vi "App - RUS scan V2.vi"(0 "Lock-in DAQ settings":T5={"Lockin mode"=enum."NI-DAQ", "DAQmx Device"="Dev2", "SR Lockin"="GPIB0::10::INSTR", "Clock Multiplier"=64, "Low-pass filter"=enum."No filtering", "Ranges and couplings "=[{"Range"=2.5, "Coupling"=10106}], "Samples per read"=20, "Record IF"=FALSE, "Auto-phase"=FALSE} {"Ranges and couplings"."Coupling" items=["default"=-1, "RSE"=10083, "NRSE"=10078, "Differential"=10106, "Pseudodifferential"=12529]}, 1 "Save data settings":T6={"Save data"=TRUE, "Data Root Path"=path "D:/Technique/RUS/CeCu2Si2/A116/2_cooling", "File Prefix"="28.49800K_100_3000_0.51000V_0.00000T_Dec19-2014__14-14-48_", "File Format"=enum."BINARY", "Save column names"=FALSE, "File Comments"="\r\nColumns:Frequency\\tX\\tY\r\n    ITC Temp= 299.200000\r\n    LTC Temp= 0.000000\r\n          ITC_set=295.00000\r\n", "User/Prj"="<User Name/Project Description>"}, 5 "temperature":dbl=28.498, 7 "sweep settings":T1={"time gap (min) "=0.0, "Bypass error dialog"=TRUE, "range factor"=1.2, "min gamma(kHz)"=0.005, "max step(Hz)"=1500.0, "min step(Hz)"=0.001, "save freq units"=enum."kHz", "Zero signal?"=FALSE, "time in Gamma --OK"=TRUE, "scan mode"=enum."peak position is known", "power control mode "=enum."none", "time-in-gamma mode"=enum."same for all"}, 9 "Fast swep settings":T4={"Update rate (Hz)"=200.0, "Start F, Hz"=100000.0, "Stop F"=3000000.0, "Number of points"=11520, "Amplitude"=0.51, "Init&amplitude"=TRUE, "IF"=1000.0, "Time constant"=0.001} {"IF" format="%#_6p"; "Amplitude" min=0.0 max=2.5; "Number of points" format="%.0p"; "Stop F" format="%#_6p"; "Start F, Hz" format="%#_6p"; "Update rate (Hz)" format="%0.2f"}, 11 "error in (no error)":errorcluster) -> (6 "Actual file path":path=path "D:/Technique/RUS/CeCu2Si2/A116/2_cooling/December_2014/121914/28.49900K_100_3000_0.51000V_0.00000T_Dec19-2014__14-13-48_001_121914.bin", 15 "error out":errorcluster)   [LabVIEW 2015]
uses:
  RUS/Controls/Sweep settings.ctl
  File/Controls/Save data settings.ctl
  File/Controls/File formats.ctl
  RUS/Controls/Lock-in DAQ settings.ctl
  single sweep - frequency chunks.ctl
  single sweep - adaptive parameters.ctl
  next chunk -- parameters.ctl
  time in gamma mode control.ctl
  find peak -- parameters.ctl
  wavepacket.ctl
  adaptive sweep UI controls.ctl
  next chunk -- algorithm.ctl
  cursor action.ctl
  four-corner circle transformation.ctl
  circle corners.ctl
  next chunk -- action.ctl
  <vilib>/Utility/error.llb/DialogType.ctl
  circle center from three points.vi
  draw a line.vi
  draw a circle.vi
  peak -- guess at omega -- dzdomega.vi
  tale of three indices.vi
  Q -- check range -- i -- real.vi
  filter -- window span logic.vi
  linear interp iiii- complex - z-omega - divide.vi
  linear interpolation iiii- complex.vi
  containing bix.vi
  generate linear region.vi
  peak -- z center from mult phase points.vi
  peak -- estimate for lorentzian.vi
  peak -- fake phase around center.vi
  peak -- get weights.vi
  peak - fit phase around center - V1.vi
  command stack.vi
  tale of three indices -- check state.vi
  Q -- check range -- i -- integer.vi
  Q - not nan -- real.vi
  linear interp iiii- complex - z-omega.vi
  line -- complex.vi
  <vilib>/Utility/error.llb/Clear Errors.vi
  Q - not nan -- integer.vi
  <vilib>/Analysis/baseanly.llb/A x B.vi
  <vilib>/Analysis/baseanly.llb/Complex A x B.vi
  <vilib>/Analysis/Matrix/Numeric/Conversions/Array To Matrix.vi
  <vilib>/Analysis/Matrix/Numeric/Conversions/Array To Matrix - RA2.vi
  <vilib>/Analysis/baseanly.llb/Inverse Matrix.vi
  <vilib>/Analysis/baseanly.llb/Real Inverse Matrix.vi
  array - generate range.vi
  peak -- fit function -- arctan.vi
  <vilib>/gmath/NumericalOptimization/Nonlinear Curve Fit.vi
  <vilib>/gmath/NumericalOptimization/Nonlinear Curve Fit LM.vi
  <resource>/objmgr/daqmx.rc
panel:
  in  "Tab : everything":enum32{"main", "everything else", "adaptive"}(tab)
  out "near omega (kHz)":dbl=50.0
  in  "Subtract a circle?":enum16{"Yes", "No"}(ring)
  in  "complex plane scale gauge":dbl(slide)=0.012396748308571648 caption="Volts" scale=0.0001..0.5
  in  "show plot pallets":bool
  in  "highlight last # sec":dbl=5.0
  out "Plot:response":cluster{dbl[], dbl[]}[](graph)=[{array[11520 elements], array[7540 elements]}, {array[11520 elements], array[7540 elements]}, {[645.57463, 645.57463], [-0.001, 0.001]}, {[769.523, 769.523], [-0.001, 0.001]}, {[1172.39758, 1172.39758], [-0.001, 0.001]}, {[1206.75312, 1206.75312], [-0.001, 0.001]}, {[1510.64651, 1510.64651], [-0.001, 0.001]}, {[1631.67457, 1631.67457], [-0.001, 0.001]}, {[2096.82648, 2096.82648], [-0.001, 0.001]}, {[2105.06377, 2105.06377], [-0.001, 0.001]}, {[2334.70001, 2334.70001], [-0.001, 0.001]}, {[2555.28377, 2555.28377], [-0.001, 0.001]}, {[2670.63046, 2670.63046], [-0.001, 0.001]}, {[2769.74725, 2769.74725], [-0.001, 0.001]}, {[2846.85386, 2846.85386], [-0.001, 0.001]}, {[2876.29657, 2876.29657], [-0.001, 0.001]}, {[2968.3015, 2968.3015], [-0.001, 0.001]}, {[2979.55486, 2979.55486], [-0.001, 0.001]}]
  out "Plot:complex plane":cluster{dbl[], dbl[]}[](graph)=[{array[7540 elements], array[7540 elements]}, {array[1000 elements], array[1000 elements]}, {[0.005000003045536789, 0.004940547817909086, 0.004763119779482496, 0.004470517076413378, 0.004067354228121515, 0.0035599893535622827, 0.0029564238998925634, 0.0022661764548692546, 0.0015001326330342118, 0.0006703734030701707, -0.00021001543629219814, -0.0011271496271373508, -0.0020665654154062474, -0.003013447652938098, -0.003952863441206996, -0.004869997632052148, -0.005750386471414516, -0.0065801457013785584, -0.0073461895232136, -0.008036436968236908, -0.008640002421906627, -0.009147367296465859, -0.009550530144757723, -0.00984313284782684, -0.010020560886253431, -0.010080016113881134, -0.010020560886253431, -0.00984313284782684, -0.009550530144757721, -0.009147367296465859, -0.008640002421906625, -0.008036436968236908, -0.007346189523213599, -0.006580145701378555, -0.005750386471414511, -0.004869997632052148, -0.003952863441206995, -0.0030134476529380966, -0.0020665654154062444, -0.0011271496271373462, -0.00021001543629219988, 0.0006703734030701703, 0.0015001326330342135, 0.0022661764548692572, 0.002956423899892566, 0.0035599893535622853, 0.004067354228121515, 0.004470517076413378, 0.004763119779482496, 0.004940547817909086], [0.00047076259399639255, 0.0014157763757271474, 0.0023458867255961384, 0.0032464252477649408, 0.004103189911783316, 0.004902669027093289, 0.0056322543304607505, 0.00628043982581846, 0.006837003240697381, 0.007293167237570003, 0.007641737837706482, 0.007877217874516685, 0.007995893687151154, 0.007995893687151154, 0.007877217874516684, 0.007641737837706482, 0.0072931672375700024, 0.00683700324069738, 0.00628043982581846, 0.005632254330460749, 0.0049026690270932895, 0.004103189911783315, 0.003246425247764939, 0.002345886725596139, 0.0014157763757271461, 0.0004707625939963901, -0.00047425118773436253, -0.0014043615376033549, -0.0023049000597721585, -0.0031616647237905308, -0.0039611438391005055, -0.004690729142467966, -0.005338914637825676, -0.005895478052704598, -0.00635164204957722, -0.0067002126497136974, -0.0069356926865239, -0.007054368499158369, -0.007054368499158369, -0.006935692686523899, -0.006700212649713698, -0.006351642049577218, -0.005895478052704595, -0.0053389146378256735, -0.004690729142467962, -0.0039611438391004995, -0.0031616647237905303, -0.002304900059772155, -0.001404361537603351, -0.00047425118773435874]}, {[-0.0036773228927567273, -0.003563591256898272, -0.0034498596210398164, -0.003336127985181361, -0.0032223963493229054, -0.0031086647134644495, -0.0029949330776059945, -0.0028812014417475386, -0.002767469805889083, -0.0026537381700306277, -0.0025400065341721722, -0.0024262748983137168, -0.0023125432624552613, -0.002198811626596806, -0.00208507999073835, -0.001971348354879895, -0.0018576167190214393, -0.0017438850831629838, -0.0016301534473045281, -0.0015164218114460727], [0.00792450366560593, 0.007179129558444975, 0.006433755451284022, 0.005688381344123069, 0.004943007236962115, 0.004197633129801161, 0.0034522590226402083, 0.0027068849154792546, 0.001961510808318301, 0.001216136701157347, 0.0004707625939963933, -0.00027461151316456045, -0.0010199856203255125, -0.0017653597274864662, -0.00251073383464742, -0.0032561079418083737, -0.0040014820489693275, -0.004746856156130281, -0.005492230263291235, -0.006237604370452189]}, {[0.004913734537437363, 0.004168360430276409, 0.003422986323115456, 0.0026776122159545028, 0.001932238108793549, 0.0011868640016325952, 0.00044148989447164236, -0.0003038842126893114, -0.0010492583198502652, -0.001794632427011219, -0.0025400065341721727, -0.0032853806413331264, -0.0040307547484940785, -0.004776128855655032, -0.005521502962815986, -0.00626687706997694, -0.0070122511771378935, -0.007757625284298847, -0.008502999391459801, -0.009248373498620755], [0.0016080789525809475, 0.001494347316722492, 0.0013806156808640366, 0.001266884045005581, 0.0011531524091471254, 0.00103942077328867, 0.0009256891374302145, 0.0008119575015717589, 0.0006982258657133035, 0.0005844942298548479, 0.00047076259399639244, 0.000357030958137937, 0.00024329932227948152, 0.00012956768642102606, 1.5836050562570382e-05, -9.789558529588508e-05, -0.00021162722115434054, -0.000325358857012796, -0.0004390904928712517, -0.0005528221287297071]}]
  in  "progress (sec)":dbl(slide)=47.30199999999604 caption="seconds" min=80.0 max=80.0 scale=0.0..54.0
  in  "Plot when running":bool
  in  "Graph update rate, ms":u32=50
  out "near gamma (kHz)":dbl=50.0
  in  "stop":bool
  out "Progress, %":u8(slide)=82 scale=0.0..100.0
  in  "Tab : sweep controls":enum32{"Main controls", "File", "Advanced"}(tab)
  in  "Manual\nPhase":dbl(slide) scale=-180.0..180.0
  out "Error status byte\n(bit 5 - FAST aborted)":u8 format="%08b"
  out "STD status byte":u8 format="%08b"
  out "DO array  making time":u32
  out "DO write time, ms":u32=23
  out "Loop counter":i32=575
  out "Pre-sweep delay, s":dbl=0.2
  out "Samples in buffer":u32
  out "Actual setup time, ms":u32=1812
  out "line two":cluster{dbl[], dbl[]}={[0.004913734537437363, 0.004168360430276409, 0.003422986323115456, 0.0026776122159545028, 0.001932238108793549, 0.0011868640016325952, 0.00044148989447164236, -0.0003038842126893114, -0.0010492583198502652, -0.001794632427011219, -0.0025400065341721727, -0.0032853806413331264, -0.0040307547484940785, -0.004776128855655032, -0.005521502962815986, -0.00626687706997694, -0.0070122511771378935, -0.007757625284298847, -0.008502999391459801, -0.009248373498620755], [0.0016080789525809475, 0.001494347316722492, 0.0013806156808640366, 0.001266884045005581, 0.0011531524091471254, 0.00103942077328867, 0.0009256891374302145, 0.0008119575015717589, 0.0006982258657133035, 0.0005844942298548479, 0.00047076259399639244, 0.000357030958137937, 0.00024329932227948152, 0.00012956768642102606, 1.5836050562570382e-05, -9.789558529588508e-05, -0.00021162722115434054, -0.000325358857012796, -0.0004390904928712517, -0.0005528221287297071]}
  out "circle":cluster{dbl[], dbl[]}={[0.005000003045536789, 0.004940547817909086, 0.004763119779482496, 0.004470517076413378, 0.004067354228121515, 0.0035599893535622827, 0.0029564238998925634, 0.0022661764548692546, 0.0015001326330342118, 0.0006703734030701707, -0.00021001543629219814, -0.0011271496271373508, -0.0020665654154062474, -0.003013447652938098, -0.003952863441206996, -0.004869997632052148, -0.005750386471414516, -0.0065801457013785584, -0.0073461895232136, -0.008036436968236908, -0.008640002421906627, -0.009147367296465859, -0.009550530144757723, -0.00984313284782684, -0.010020560886253431, -0.010080016113881134, -0.010020560886253431, -0.00984313284782684, -0.009550530144757721, -0.009147367296465859, -0.008640002421906625, -0.008036436968236908, -0.007346189523213599, -0.006580145701378555, -0.005750386471414511, -0.004869997632052148, -0.003952863441206995, -0.0030134476529380966, -0.0020665654154062444, -0.0011271496271373462, -0.00021001543629219988, 0.0006703734030701703, 0.0015001326330342135, 0.0022661764548692572, 0.002956423899892566, 0.0035599893535622853, 0.004067354228121515, 0.004470517076413378, 0.004763119779482496, 0.004940547817909086], [0.00047076259399639255, 0.0014157763757271474, 0.0023458867255961384, 0.0032464252477649408, 0.004103189911783316, 0.004902669027093289, 0.0056322543304607505, 0.00628043982581846, 0.006837003240697381, 0.007293167237570003, 0.007641737837706482, 0.007877217874516685, 0.007995893687151154, 0.007995893687151154, 0.007877217874516684, 0.007641737837706482, 0.0072931672375700024, 0.00683700324069738, 0.00628043982581846, 0.005632254330460749, 0.0049026690270932895, 0.004103189911783315, 0.003246425247764939, 0.002345886725596139, 0.0014157763757271461, 0.0004707625939963901, -0.00047425118773436253, -0.0014043615376033549, -0.0023049000597721585, -0.0031616647237905308, -0.0039611438391005055, -0.004690729142467966, -0.005338914637825676, -0.005895478052704598, -0.00635164204957722, -0.0067002126497136974, -0.0069356926865239, -0.007054368499158369, -0.007054368499158369, -0.006935692686523899, -0.006700212649713698, -0.006351642049577218, -0.005895478052704595, -0.0053389146378256735, -0.004690729142467962, -0.0039611438391004995, -0.0031616647237905303, -0.002304900059772155, -0.001404361537603351, -0.00047425118773435874]}
  out "line one":cluster{dbl[], dbl[]}={[-0.0036773228927567273, -0.003563591256898272, -0.0034498596210398164, -0.003336127985181361, -0.0032223963493229054, -0.0031086647134644495, -0.0029949330776059945, -0.0028812014417475386, -0.002767469805889083, -0.0026537381700306277, -0.0025400065341721722, -0.0024262748983137168, -0.0023125432624552613, -0.002198811626596806, -0.00208507999073835, -0.001971348354879895, -0.0018576167190214393, -0.0017438850831629838, -0.0016301534473045281, -0.0015164218114460727], [0.00792450366560593, 0.007179129558444975, 0.006433755451284022, 0.005688381344123069, 0.004943007236962115, 0.004197633129801161, 0.0034522590226402083, 0.0027068849154792546, 0.001961510808318301, 0.001216136701157347, 0.0004707625939963933, -0.00027461151316456045, -0.0010199856203255125, -0.0017653597274864662, -0.00251073383464742, -0.0032561079418083737, -0.0040014820489693275, -0.004746856156130281, -0.005492230263291235, -0.006237604370452189]}
  out "frequency":dbl[](array[numeric])
  out "complex data":cdb[](array[numeric])
  out "#data points so far":i32=9480
  out "last data":cdb[](array[numeric])=[-0.0013862457351888618+0.00908142415858101i, -0.0013023312189548073+0.009148157349497919i, -0.001321430292511047+0.009061460065413475i, -0.001363391573336929+0.009045433130201685i, -0.001296708698532554+0.009000112664646402i, -0.0013667002669505222+0.009050113974772414i, -0.0012817676519993981+0.009066319936344113i, -0.0013424252885312644+0.008962242292230364i, -0.0014137356567434898+0.009049299475543717i, -0.0012869072704579012+0.00899110197613083i, -0.0013910227339383506+0.009040086299077377i, -0.0013472731057654439+0.009083303189564951i, -0.001381966900473036+0.009046535653865845i, -0.0013652417984066345+0.009101756771060749i, -0.0013461643267386587+0.008999329508834603i, -0.0013471376638622685+0.009069385579497309i, -0.0013236258377476435+0.009072036195700378i, -0.0013196021377368792+0.009075087400102249i, -0.0013182324903640112+0.009113697088335707i, -0.0012918150838322992+0.009064845988581937i]
  out "fancy circles":cluster{dbl[], dbl[]}[](array[cluster])
  out "fancy lines":cluster{dbl[], dbl[]}[](array[cluster])=[{[645.57463, 645.57463], [-0.001, 0.001]}, {[769.523, 769.523], [-0.001, 0.001]}, {[1172.39758, 1172.39758], [-0.001, 0.001]}, {[1206.75312, 1206.75312], [-0.001, 0.001]}, {[1510.64651, 1510.64651], [-0.001, 0.001]}, {[1631.67457, 1631.67457], [-0.001, 0.001]}, {[2096.82648, 2096.82648], [-0.001, 0.001]}, {[2105.06377, 2105.06377], [-0.001, 0.001]}, {[2334.70001, 2334.70001], [-0.001, 0.001]}, {[2555.28377, 2555.28377], [-0.001, 0.001]}, {[2670.63046, 2670.63046], [-0.001, 0.001]}, {[2769.74725, 2769.74725], [-0.001, 0.001]}, {[2846.85386, 2846.85386], [-0.001, 0.001]}, {[2876.29657, 2876.29657], [-0.001, 0.001]}, {[2968.3015, 2968.3015], [-0.001, 0.001]}, {[2979.55486, 2979.55486], [-0.001, 0.001]}]
  in  "adaptive state":T8={"peaks are known -- parameters"={"Def Gamma (kHz)"=10.0, "dV"=17.0, "time in Gamma (sec)"=3.0, "phi-star"=0.0, "all peaks (kHz)"=[645.57463, 769.523, 1172.39758, 1206.75312, 1510.64651, 1631.67457, 2096.82648, 2105.06377, 2334.70001, 2555.28377, 2670.63046, 2769.74725, 2846.85386, 2876.29657, 2968.3015, 2979.55486], "delta t (sec)"=0.005, "default step (Hz)"=251.73611111111111, "all gamma (kHz)"=[0.05963, 1.26052, 0.07474, 0.14496, 0.02522, 0.0921, 0.08571, 0.32008, 0.01, 0.00491, 2.14403, 0.17331, 7.48912, 0.20157, 0.17918, 0.145], "peaks OK"=TRUE, "gamma OK"=TRUE, "near omega (kHz)"=0.0, "near gamma (kHz)"=0.0, "min step (Hz)"=0.001, "max step(Hz)"=1500.0, "min gamma (kHz)"=0.005, "all time in gamma (sec)"=[], "time in gamma OK"=FALSE, "time-in-gamma mode"=enum."same for all"}, "find peak - parameters"={"wavepacket"={"R"=0.5, "wave number"=17.0, "delta k"=7.0, "radii vector"=[], "radial section"=[], "wave vector"=22.0, "wavepacket is"=TRUE}, "number of grid points"=70, "decimation threshold"=1, "Voltage range"=0.1, "target freq step"=20.0, "target spot size"=0.05, "factor"=1.0, "another factor"=1.0, "analyze last # sec"=3, "scale factor"=3}} {"find peak - parameters"."wavepacket"."delta k" format="%#_3f"; "find peak - parameters"."wavepacket"."wave number" format="%#_3f"; "find peak - parameters"."wavepacket"."R" format="%#_3f"}
  in  "chunks":T12={"start F (Hz)"=100000.0, "stop F (Hz)"=3000000.0, "total number of points"=11520, "chunk size"=20, "freq step (Hz)"=0.7518687555352066, "update rate (Hz)"=200.0, "adaptive parameters"={"peaks are known -- parameters"={"Def Gamma (kHz)"=10.0, "dV"=17.0, "time in Gamma (sec)"=3.0, "phi-star"=0.0, "all peaks (kHz)"=[645.57463, 769.523, 1172.39758, 1206.75312, 1510.64651, 1631.67457, 2096.82648, 2105.06377, 2334.70001, 2555.28377, 2670.63046, 2769.74725, 2846.85386, 2876.29657, 2968.3015, 2979.55486], "delta t (sec)"=0.005, "default step (Hz)"=251.73611111111111, "all gamma (kHz)"=[0.05963, 1.26052, 0.07474, 0.14496, 0.02522, 0.0921, 0.08571, 0.32008, 0.01, 0.00491, 2.14403, 0.17331, 7.48912, 0.20157, 0.17918, 0.145], "peaks OK"=TRUE, "gamma OK"=TRUE, "near omega (kHz)"=0.0, "near gamma (kHz)"=0.0, "min step (Hz)"=0.001, "max step(Hz)"=1500.0, "min gamma (kHz)"=0.005, "all time in gamma (sec)"=[], "time in gamma OK"=FALSE, "time-in-gamma mode"=enum."same for all"}, "find peak - parameters"={"wavepacket"={"R"=0.5, "wave number"=17.0, "delta k"=7.0, "radii vector"=[], "radial section"=[], "wave vector"=22.0, "wavepacket is"=TRUE}, "number of grid points"=70, "decimation threshold"=1, "Voltage range"=0.1, "target freq step"=20.0, "target spot size"=0.05, "factor"=1.0, "another factor"=1.0, "analyze last # sec"=3, "scale factor"=3}}, "total sweep time (sec)"=57.6, "chunk time (sec)"=0.1, "spot size (V)"=0.0, "uniform freq step (Hz)"=251.73611111111111, "next start freq (Hz)"=2876231.1242983374} {"next start freq (Hz)" format="%#9_8f"; "uniform freq step (Hz)" format="%#_3f"; "spot size (V)" format="%#_2f"; "adaptive parameters"."find peak - parameters"."wavepacket"."delta k" format="%#_3f"; "adaptive parameters"."find peak - parameters"."wavepacket"."wave number" format="%#_3f"; "adaptive parameters"."find peak - parameters"."wavepacket"."R" format="%#_3f"; "freq step (Hz)" format="%#4_4f"; "stop F (Hz)" format="%#_3f"; "start F (Hz)" format="%#_3f"}
  # "SRS Lockin related"
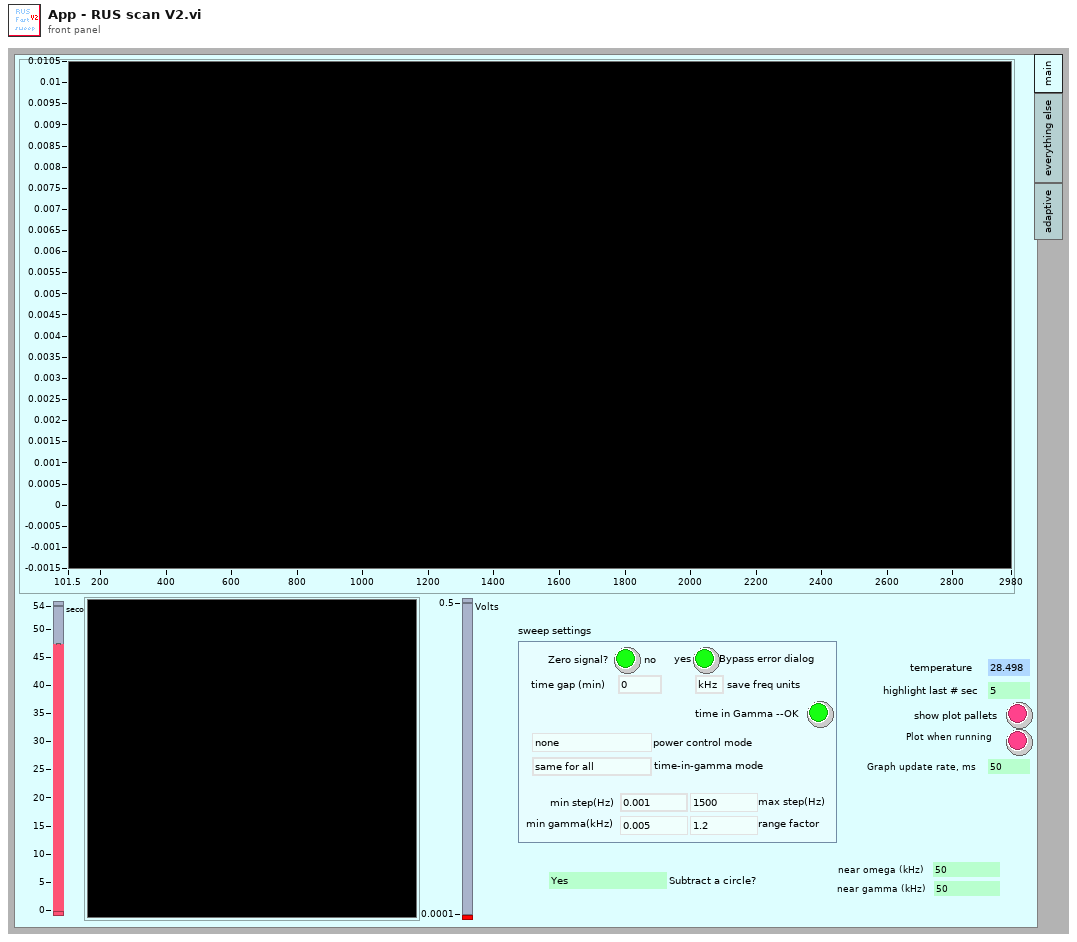
[diagram p1: front panel]
types:
  T1 = typedef "adaptive sweep UI controls.ctl" = cluster{"time gap (min) ":dbl, "Bypass error dialog":bool, "range factor":dbl, "min gamma(kHz)":dbl, "max step(Hz)":dbl, "min step(Hz)":dbl, "save freq units":enum16{"kHz", "Hz"}, "Zero signal?":bool, "time in Gamma --OK":bool, "scan mode":T2, "power control mode ":enum16{"power vs Temp", "power vs Time", "none"}, "time-in-gamma mode":T3}
  T2 = typedef "next chunk -- algorithm.ctl" = enum16{"peak position is known", "uniform", "predictive"}
  T3 = typedef "time in gamma mode control.ctl" = enum16{"same for all", "each one different", "uniform scan"}
  T4 = typedef "Sweep settings.ctl" = cluster{"Update rate (Hz)":dbl, "Start F, Hz":dbl, "Stop F":dbl, "Number of points":i32, "Amplitude":dbl, "Init&amplitude":bool, "IF":dbl, "Time constant":dbl}
  T5 = typedef "Lock-in DAQ settings.ctl" = cluster{"Lockin mode":enum16{"SRS", "NI-DAQ"}, "DAQmx Device":tag, "SR Lockin":refnum<visa-resource-name>, "Clock Multiplier":i32, "Low-pass filter":enum16{"No filtering", "Butterworth", "Bessel"}, "Ranges and couplings ":cluster{"Range":dbl, "Coupling":i32}[], "Samples per read":i32, "Record IF":bool, "Auto-phase":bool}
  T6 = typedef "Save data settings.ctl" = cluster{"Save data":bool, "Data Root Path":path, "File Prefix":string, "File Format":T7, "Save column names":bool, "File Comments":string, "User/Prj":string}
  T7 = typedef "File formats.ctl" = enum16{"TDMS", "ASCII", "BINARY"}
  T8 = typedef "single sweep - adaptive parameters.ctl" = cluster{"peaks are known -- parameters":T9, "find peak - parameters":T10}
  T9 = typedef "next chunk -- parameters.ctl" = cluster{"Def Gamma (kHz)":dbl, "dV":dbl, "time in Gamma (sec)":dbl, "phi-star":dbl, "all peaks (kHz)":dbl[], "delta t (sec)":dbl, "default step (Hz)":dbl, "all gamma (kHz)":dbl[], "peaks OK":bool, "gamma OK":bool, "near omega (kHz)":dbl, "near gamma (kHz)":dbl, "min step (Hz)":dbl, "max step(Hz)":dbl, "min gamma (kHz)":dbl, "all time in gamma (sec)":dbl[], "time in gamma OK":bool, "time-in-gamma mode":T3}
  T10 = typedef "find peak -- parameters.ctl" = cluster{"wavepacket":T11, "number of grid points":i32, "decimation threshold":i32, "Voltage range":dbl, "target freq step":dbl, "target spot size":dbl, "factor":dbl, "another factor":dbl, "analyze last # sec":i32, "scale factor":i32}
  T11 = typedef "wavepacket.ctl" = cluster{"R":dbl, "wave number":dbl, "delta k":dbl, "radii vector":dbl[], "radial section":cdb[], "wave vector":dbl, "wavepacket is":bool}
  T12 = typedef "single sweep - frequency chunks.ctl" = cluster{"start F (Hz)":dbl, "stop F (Hz)":dbl, "total number of points":i32, "chunk size":i32, "freq step (Hz)":dbl, "update rate (Hz)":dbl, "adaptive parameters":T8, "total sweep time (sec)":dbl, "chunk time (sec)":dbl, "spot size (V)":dbl, "uniform freq step (Hz)":dbl, "next start freq (Hz)":dbl}
  T13 = typedef "RUS settings.ctl" = cluster{"NI-DAQ lockin settings":T14, "Fast swep settings":T4, "Pre-sweep delay, s":dbl, "Lockin mode":enum16{"SRS", "NI-DAQ"}, "SR Lockin":refnum<visa-resource-name>, "DAQmx Device":tag, "Clock Multiplier":i32, "Fast Sweep Data Out":cluster{"DO clock task":refnum<k21>, "DO task":refnum<k21>, "Update clock task":refnum<k21>, "DAQ lockin task":refnum<k21>, "Pre-sweep counter task":refnum<k21>}, "Lockin Range, V":sgl, "F Array":dbl[], "Freq. update clock terminal":string, "DO Clock Rate (Hz)":dbl, "ADC clock terminal":string, "Pre-sweep counter terminal":string, "Samples per read":i32, "DO clock terminal":string, "Pre-sweep points":i32, "F points per write":i32, "Total sweep time, s":dbl, "Initial SYNTH phase":dbl, "Record IF":bool, "Save data settings":T6, "Data file path":path, "New data user event":refnum<user-event>, "Stop user event":refnum<user-event>, "Number of channels":i32, "Auto-phase":bool}
  T14 = typedef "RUS NI-DAQ Lockin Settings.ctl" = cluster{"Samples per sine wave":i32, "Sine waves per freq step":i32, "Output Representation":enum16{"Real/Imaginary", "Polar"}, "Low-pass filter":enum16{"No filtering", "Butterworth", "Bessel"}, "Ranges and couplings ":cluster{"Range":dbl, "Coupling":i32}[]}
  T15 = typedef "next chunk -- action.ctl" = enum16{"empty", "init - uniform", "next chunk - uniform", "next chunk - peaks are known", "init - peaks are known", ""}
  T16 = typedef "circle corners.ctl" = cluster{"z (-pi/2)":cdb, "z(inf)":cdb, "z (pi/2)":cdb, "z center":cdb, "z(0)":cdb, "radius":dbl}
  T17 = typedef "four-corner circle transformation.ctl" = enum16{"z(c) z(inf)", "z(c) z(zero)", "fix phase", "calculate lorentzian", "z(0) z(+-pi/2)", "shift to zcenter"}
  T18 = typedef "cursor action.ctl" = enum16{"range", "read", "write", "check", "zoom out", "smart zoom out"}
  T19 = typedef "DialogType.ctl" = u16
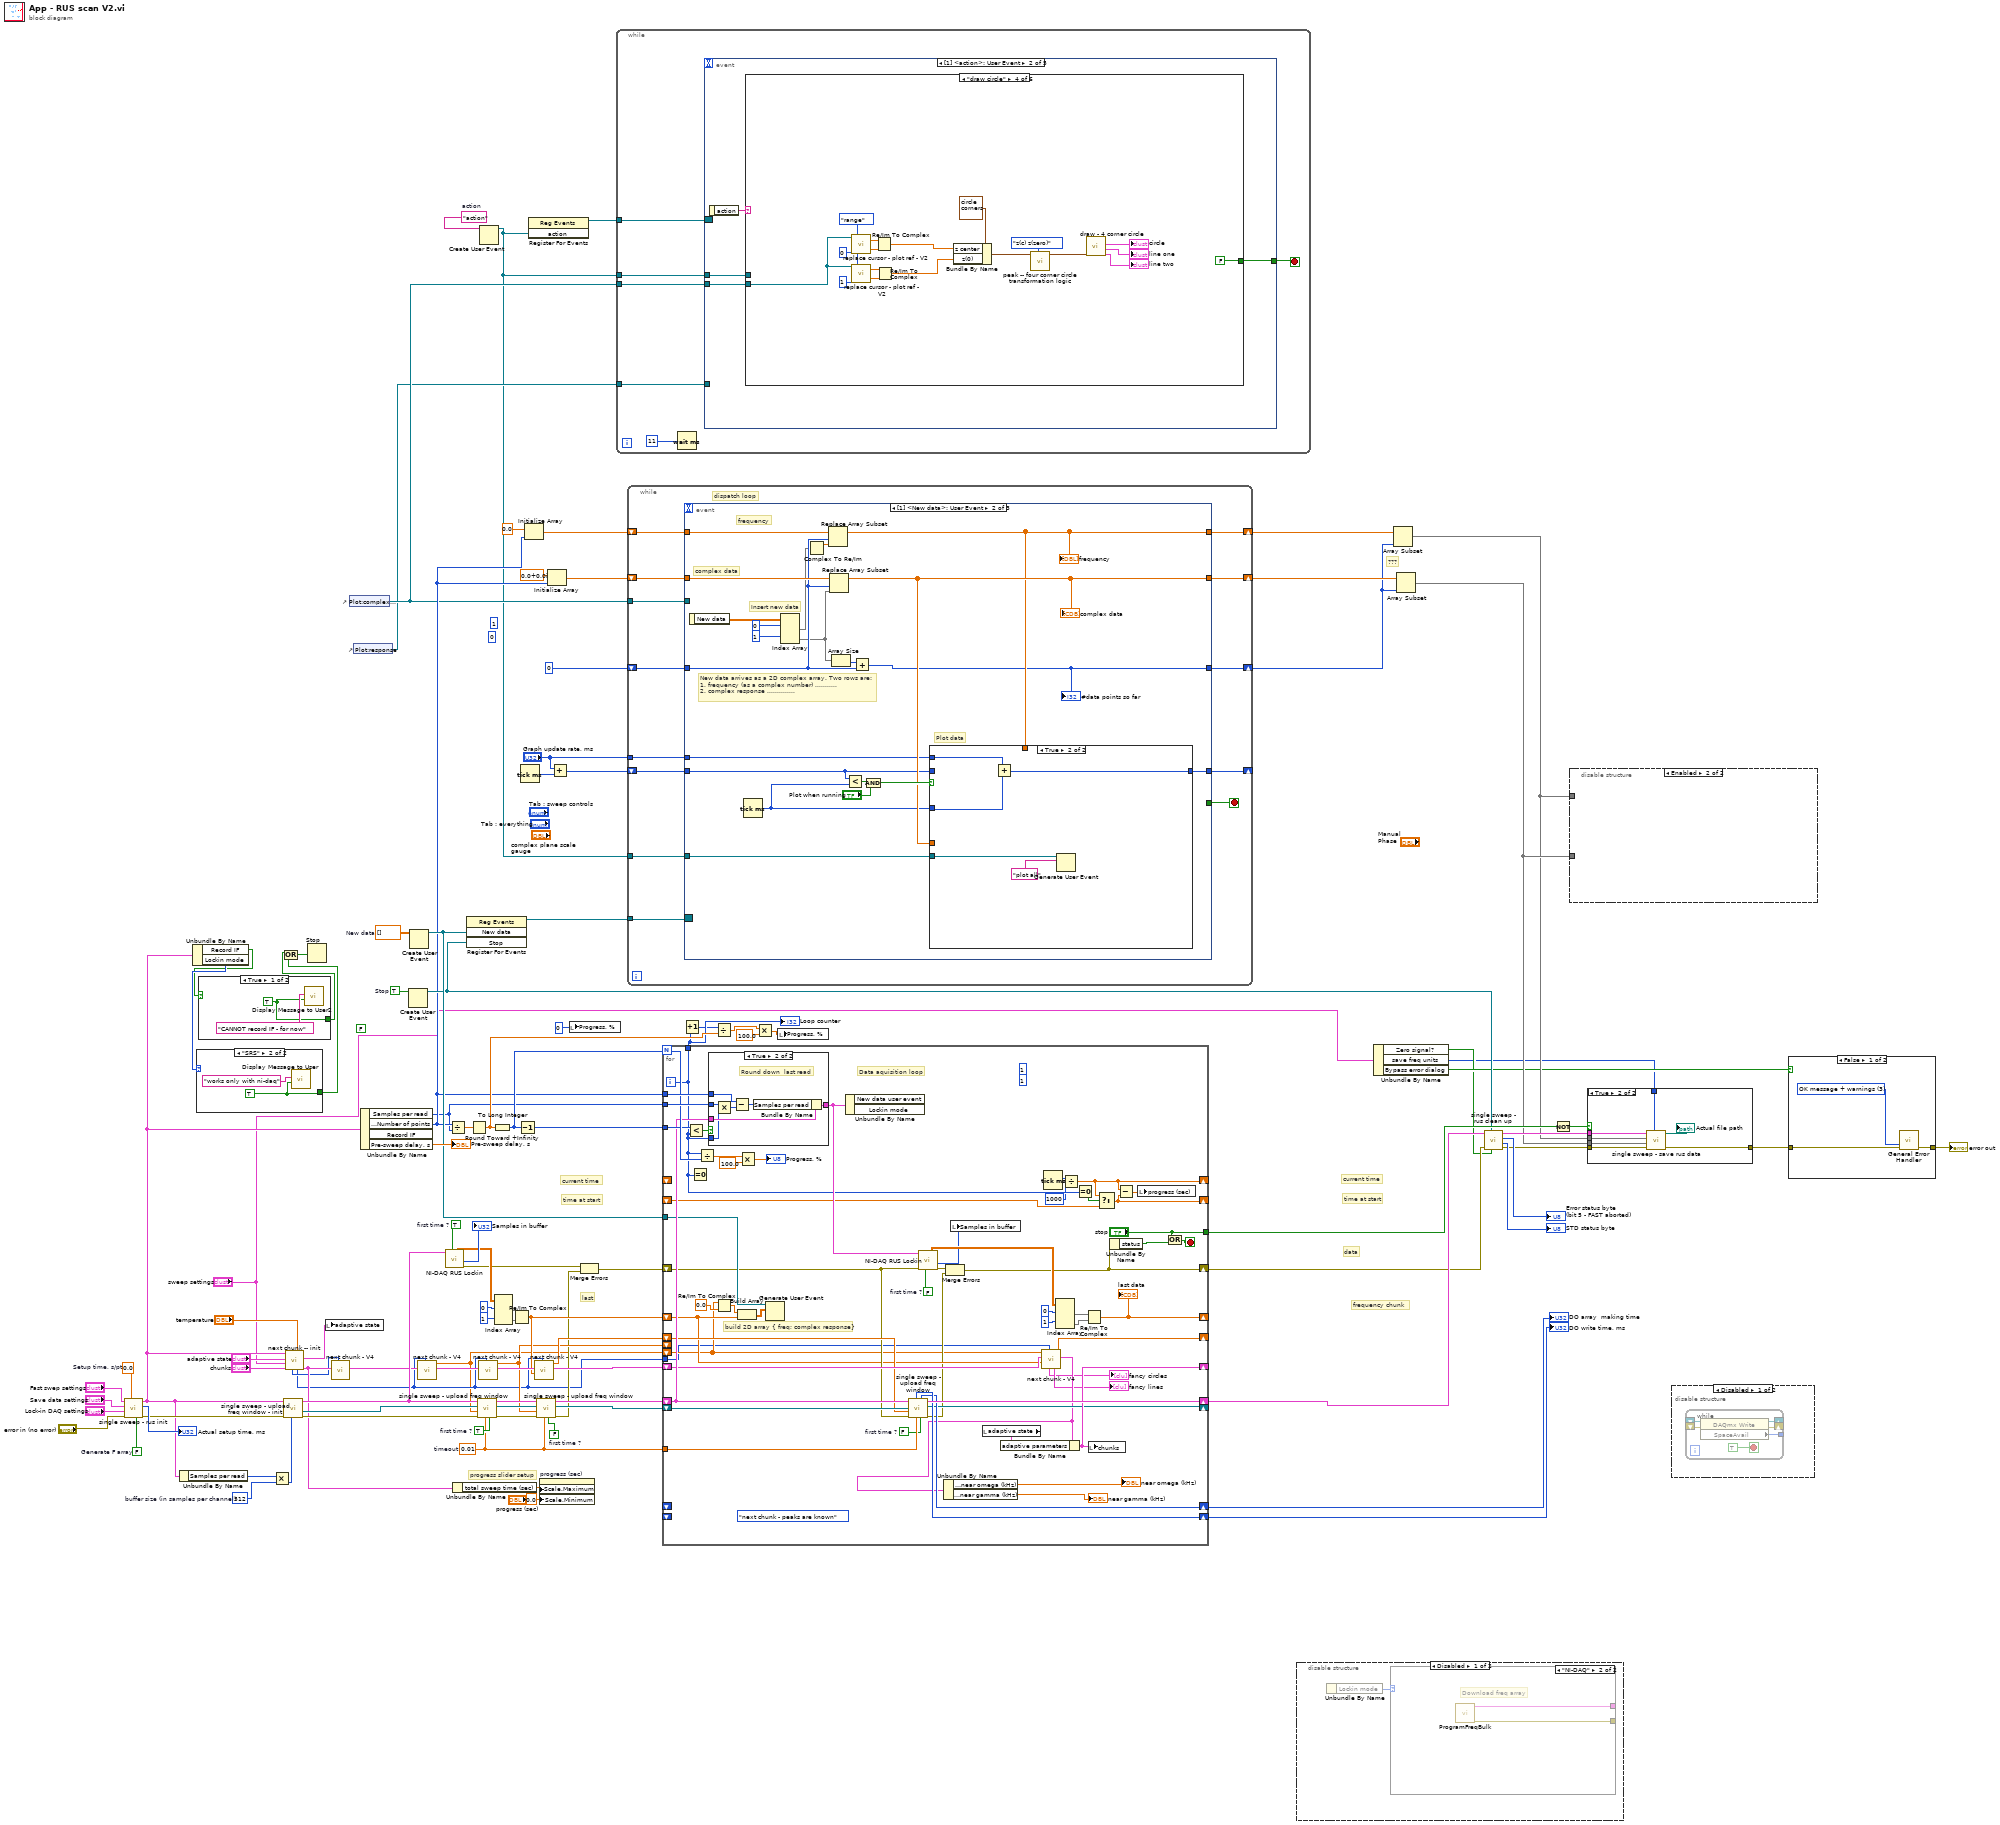
[diagram p0: block diagram]
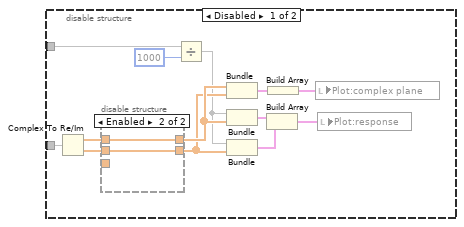
[diagram p2: hidden frame]
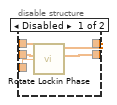
[diagram p3: hidden frame]
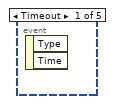
[diagram p4: hidden frame]
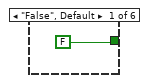
[diagram p5: hidden frame]
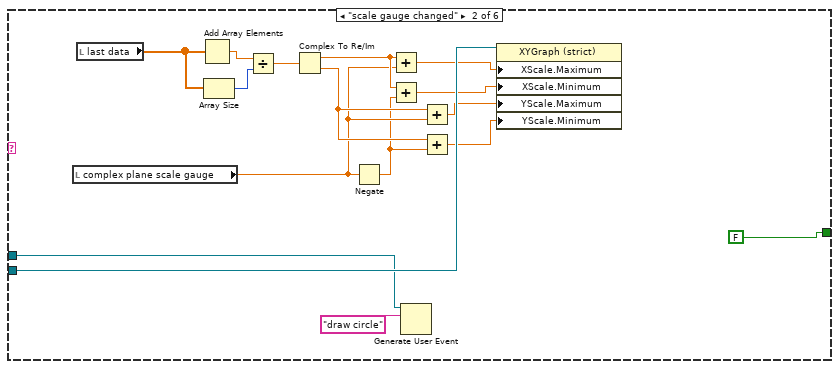
[diagram p6: hidden frame]
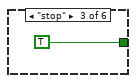
[diagram p7: hidden frame]
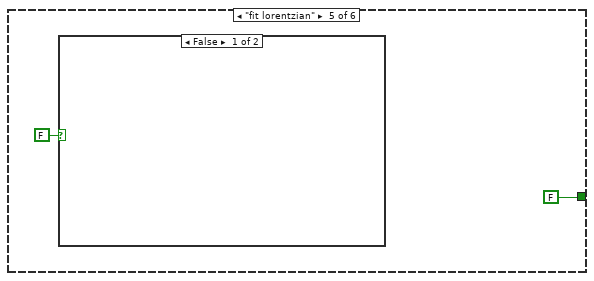
[diagram p8: hidden frame]
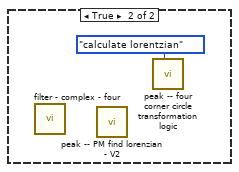
[diagram p9: hidden frame]
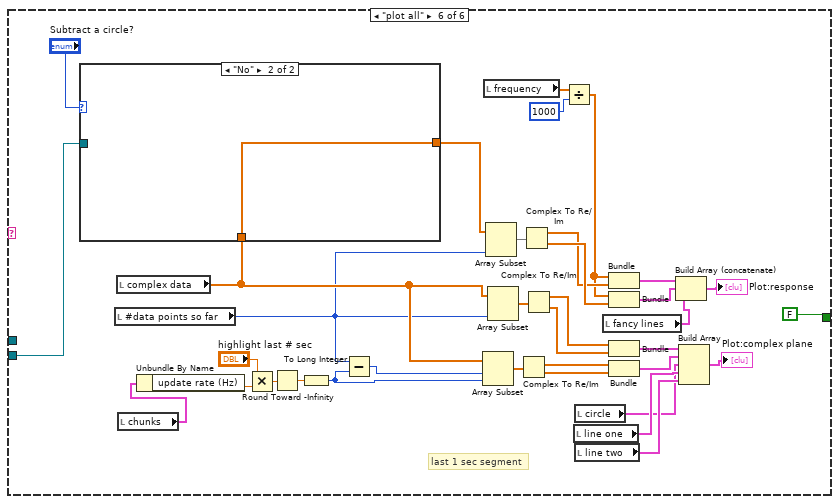
[diagram p10: hidden frame]
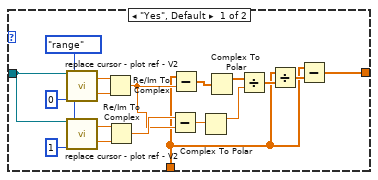
[diagram p11: hidden frame]
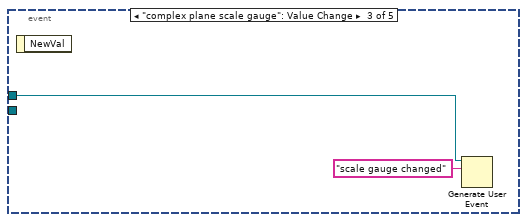
[diagram p12: hidden frame]
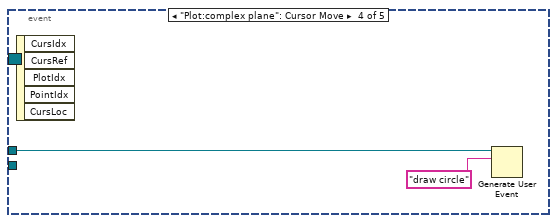
[diagram p13: hidden frame]
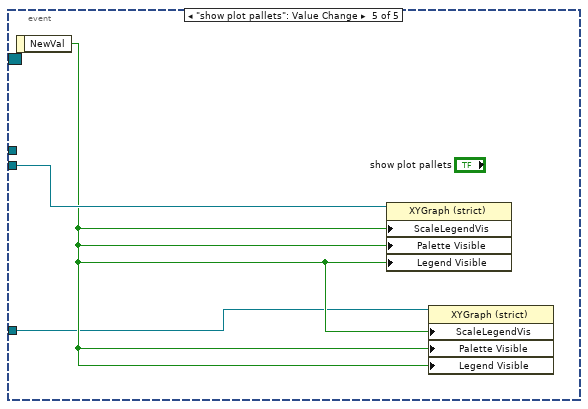
[diagram p14: hidden frame]
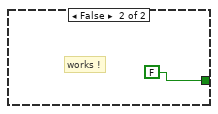
[diagram p16: hidden frame]
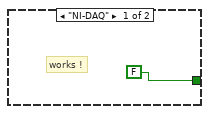
[diagram p17: hidden frame]
diagram:
  w5 = "action"  # action
  w28 = TRUE  # first time ?
  w29 = FALSE  # Generate F array
  w30 = 0.0  # Setup time, s/pt
  w33 = u32 512  # buffer size (in samples per channel)
  w48 = FALSE  # first time ?
  (unwired) 0 ("disabled index (col)")
  (unwired) FALSE
  (unwired) 1 ("dimension size")
  w67 = cdb[][] []  # New data
  w69 = TRUE  # Stop
  w73 = TRUE  # first time ?
  w41 = 0.01  # timeout
  # "data"
  # "frequency chunk"
  # "last"
  # "time at start"
  # "current time"
  # "time at start"
  # "current time"
  # "progress slider setup"
  # "???"
  n1 = call "single sweep - rus init.vi"("Generate F array"=w29, "Setup time, s/pt"=w30, "error in (no error)"="error in (no error)", "Lock-in DAQ settings"="Lock-in DAQ settings", "Save data settings"="Save data settings", "Fast swep settings"="Fast swep settings") -> ("error out"=w76:errorcluster, "Actual setup time, ms"=→"Actual setup time, ms":u32, "RUS settings out"=w18:T13)  [unwired: 2 in, 1 out]
  n2 = Unbundle By Name(w18) -> ("Samples per read"=w31:i32)
  n3 = Unbundle By Name(w18) -> ("Record IF"=w56:bool, "Lockin mode"=w75:enum16{"SRS", "NI-DAQ"})
  n4 = case shown="\"SRS\"" w75 {
    tunnel: [FALSE w108] -> w58
    frame "NI-DAQ" {
      # "works !"
    }
    frame "SRS" {
      w108 = TRUE
      n5 = call "Display Message to User"("Enable"=w108, "Message"="works only with ni-daq") -> ()  [unwired: 8 in, 2 out]
    }
  }
  n6 = case shown="True" w56 {
    tunnel: [w110 FALSE] -> w57
    frame True {
      w110 = TRUE
      n7 = call "Display Message to User2"("Enable"=w110, "Message"="CANNOT record IF - for now") -> ()  [unwired: 8 in, 2 out]
    }
    frame False {
      # "works !"
    }
  }
  n8 = Multiply(x=w31, y=w33) -> (x*y=w32:u32)
  n9 = Or(x=w57, y=w58) -> (x .or. y?=w55:bool)
  n10 = call "single sweep - upload freq window - init.vi"("buffer size (in samples per channel)"=w32, "error in (no error)"=w76, "RUS settings"=w18) -> ("error - out"=w37:errorcluster, "task out"=w74:refnum<k21>, "RUS settings out"=w49:T13)  [unwired: 6 in]
  n11 = call "next chunk -- init.vi"("temperature"="temperature", "chunks"="chunks", "sweep settings"="sweep settings", "adaptive parameters"="adaptive state", "RUS settings"=w18) -> ("chunks out"=w17:T12, "adaptive parameters out"=w15:T8, "next chunk action"=w11:T15, "next chunk init action"=w14:T15)  [unwired: 3 in]
  n12 = Stop(stop? (T)=w55) -> ()
  n13 = local write "adaptive state"(w15) -> ()
  n14 = call "next chunk - V4.vi"("next chunk action"=w14, "chunks"=w17) -> ("chunks out"=w12:T12)  [unwired: 6 in, 3 out]
  n15 = control-ref of="Plot:complex plane"() -> (w3:refnum<vi>)
  n16 = control-ref of="Plot:response"() -> (w2:refnum<vi>)
  n17 = Unbundle By Name(w18) -> ("Samples per read"=w50:i32, "Fast swep settings.Number of points"=w51:i32, "Pre-sweep delay, s"=→"Pre-sweep delay, s":dbl)  [unwired: 1 out]
  n18 = Create User Event(user event datatype=w69) -> (user event=w62:refnum<user-event>)  [unwired: 1 in, 1 out]
  n19 = Create User Event(user event datatype=w67) -> (user event=w68:refnum<user-event>)  [unwired: 1 in, 1 out]
  n20 = call "next chunk - V4.vi"("next chunk action"=w11, "chunks"=w12) -> ("F Array out"=w10:dbl[])  [unwired: 6 in, 3 out]
  n21 = call "NI-DAQ RUS Lockin.vi"("Init?"=w28, "RUS settings"=w49) -> ("error out"=w21:errorcluster, "AvailSampPerChan"=→"Samples in buffer":u32, "Lockin out"=w22:dbl[][])  [unwired: 6 in, 1 out]
  n22 = Divide(x=w51, y=w50) -> (x/y=w104:dbl)
  n23 = Unbundle By Name(w17) -> ("total sweep time (sec)"=w54:dbl)
  n24 = register-events(w68, w62) -> (reference out=w70:refnum<event-registration>)  [unwired: 2 in, 1 out]
  n25 = Round Toward +Infinity(x=w104) -> (ceil(x): smallest int >= x=w98:dbl)
  n26 = call "single sweep - upload freq window.vi"("first time ?"=w73, "timeout"=w41, "error in (no error)"=w37, "F-window array"=w10, "task in"=w74, "RUS settings"=w49) -> ("error out"=w36:errorcluster, "task out"=w44:refnum<k21>, "RUS settings out"=w47:T13)  [unwired: 1 in, 2 out]
  n27 = call "next chunk - V4.vi"("next chunk action"=w11, "chunks"=w12) -> ("chunks out"=w43:T12, "F Array out"=w34:dbl[])  [unwired: 6 in, 2 out]
  n28 = Create User Event(user event datatype=w5) -> (user event=w1:refnum<user-event>)  [unwired: 1 in, 1 out]
  n29 = To Long Integer(number=w98) -> (32bit integer=w85:i32)
  n30 = Index Array(array=w22, index (row) #1=0 ("index"), index (row) #2=1 ("length")) -> (element #1=w24:dbl[], element #2=w23:dbl[])  [unwired: 2 in]
  n31 = Re/Im To Complex(1:w23, 2:w24) -> (0:w35:cdb[])
  n32 = Decrement(x=w85) -> (x-1=w94:i32)
  n33 = Tick Count (ms)() -> (millisecond timer value=w105:u32)
  n34 = Initialize Array(0.0 ("Numeric"), w51) -> (w64:dbl[])
  n35 = register-events(w1) -> (reference out=w4:refnum<event-registration>)  [unwired: 2 in, 1 out]
  n36 = call "next chunk - V4.vi"("next chunk action"=w11, "x + iy"=w35, "chunks"=w43) -> ("chunks out"=w42:T12, "F Array out"=w39:dbl[])  [unwired: 5 in, 2 out]
  n37 = call "single sweep - upload freq window.vi"("first time ?"=w48, "timeout"=w41, "error in (no error)"=w36, "F-window array"=w34, "task in"=w44, "RUS settings"=w47) -> ("error out"=w20:errorcluster, "task out"=w45:refnum<k21>, "RUS settings out"=w46:T13)  [unwired: 1 in, 2 out]
  n38 = property on="progress (sec)" class="Slide (strict)"("Scale.Maximum"=w54, "Scale.Minimum"=0.0 ("Data Entry Limits:Minimum")) -> ()  [unwired: 2 in, 2 out]
  n39 = Initialize Array(cdb 0.0+0.0i ("Numeric"), w51) -> (w96:cdb[])
  n40 = Add(x="Graph update rate, ms", y=w105) -> (x+y=w78:u32)
  n41 = local write "Progress, %"(u8 0 ("Progress")) -> ()
  n42 = Merge Errors(w21, w20) -> (w40:errorcluster)
  n43 = while {
    tunnel: w4 -> [w117]
    tunnel: w3 -> [w116]
    tunnel: w1 -> [w115]
    tunnel: w2 -> [w114]
    stop <- w113 stop-if-true
    n44 = Wait (ms)(milliseconds to wait=u32 11) -> ()  [unwired: 1 out]
    n45 = event shown="[1] <action>: User Event" {
      selector: w117 -> [_ _ _ _ _]
      dyn-events: _ -> [_ _ _ _ _]
      timeout: _ -> [_ _ _ _ _]
      tunnel: w116 -> [_ w121 _ _ w222]
      tunnel: w115 -> [_ w120 w216 w218 _]
      tunnel: w114 -> [_ _ _ _ w220]
      tunnel: [_ w119 _ _ _] -> w113
      event Timeout {
        n46 = event-data() -> ()  [unwired: 1 in, 2 out]
      }
      event User Event {
        n47 = event-data() -> ("action"=w122:string)  [unwired: 1 in]
        n48 = case shown="\"draw circle\"" w122 {
          tunnel: w121 -> [_ w139 _ w144 _ w169]
          tunnel: w120 -> [_ w137 _ _ _ _]
          tunnel: [FALSE FALSE TRUE FALSE FALSE FALSE] -> w119
          frame "False", Default {
          }
          frame "scale gauge changed" {
            n49 = local read "complex plane scale gauge"() -> (w128:dbl)
            n50 = local read "last data"() -> (w124:cdb[])
            n51 = Add Array Elements(numeric array=w124) -> (sum=w135:cdb)
            n52 = Array Size(array=w124) -> (size(s)=w134:i32)
            n53 = Divide(x=w135, y=w134) -> (x/y=w133:cdb)
            n54 = Complex To Re/Im(x + iy=w133) -> (x=w132:dbl, y=w129:dbl)
            n55 = Negate(x=w128) -> (-x=w127:dbl)
            n56 = Add(x=w132, y=w128) -> (x+y=w131:dbl)
            n57 = Add(x=w132, y=w127) -> (x+y=w130:dbl)
            n58 = Generate User Event(user event=w137, event data cluster="draw circle" ("event data")) -> ()  [unwired: 2 in, 2 out]
            n59 = Add(x=w129, y=w128) -> (x+y=w126:dbl)
            n60 = Add(x=w129, y=w127) -> (x+y=w125:dbl)
            n61 = property on="Property Node" class="XYGraph (strict)"(reference=w139, "XScale.Maximum"=w131, "XScale.Minimum"=w130, "YScale.Maximum"=w126, "YScale.Minimum"=w125) -> ()  [unwired: 1 in, 2 out]
          }
          frame "stop" {
          }
          frame "draw circle" {
            w156 = cursor_action."range" ("cursor action")
            n62 = call "replace cursor - plot ref - V2.vi"("Plot ref in"=w144, "cursor index"=0, "cursor action"=w156) -> ("read X"=w154:dbl, "read Y"=w153:dbl)  [unwired: 14 in, 1 out]
            n63 = call "replace cursor - plot ref - V2.vi"("Plot ref in"=w144, "cursor index"=1, "cursor action"=w156) -> ("read X"=w151:dbl, "read Y"=w150:dbl)  [unwired: 14 in, 1 out]
            n64 = Re/Im To Complex(1:w153, 2:w154) -> (0:w152:cdb)
            n65 = Re/Im To Complex(1:w150, 2:w151) -> (0:w149:cdb)
            n66 = Bundle By Name(cluster=T16 {"z (-pi/2)"=-1.0311345636926572+0.5736824521422934i, "z(inf)"=-0.5200164984937075+1.0975277942502903i, "z (pi/2)"=-1.0311345636926572+0.5736824521422934i, "z center"=-0.5136528600391839+0.580046090596817i, "z(0)"=-0.5200164984937075+1.0975277942502903i, "radius"=-1.0311345636926572} ("circle corners in"), "z center"=w152, "z(0)"=w149) -> (w143:T16)
            n67 = call "peak -- four corner circle transformation logic.vi"("4 corner circle transformation"=four-corner_circle_transformation."z(c) z(zero)", "circle corners in"=w143) -> ("circle corners out"=w148:T16)  [unwired: 8 in, 1 out]
            n68 = call "draw - 4 corner circle.vi"("4corners"=w148) -> ("line two"=→"line two":cluster{dbl[], dbl[]}, "line one"=→"line one":cluster{dbl[], dbl[]}, "circle"=→"circle":cluster{dbl[], dbl[]})  [unwired: 8 in]
          }
          frame "fit lorentzian" {
            n69 = case shown="False" FALSE {
              frame False {
              }
              frame True {
                n70 = call "filter - complex - four.vi"() -> ()  [unwired: 12 in, 8 out]
                n71 = call "peak -- PM find lorenzian - V2.vi"() -> ()  [unwired: 12 in, 4 out]
                n72 = call "peak -- four corner circle transformation logic.vi"("4 corner circle transformation"=four-corner_circle_transformation."calculate lorentzian") -> ()  [unwired: 9 in, 2 out]
              }
            }
          }
          frame "plot all" {
            # "last 1 sec segment"
            n73 = local read "#data points so far"() -> (w165:i32)
            n74 = local read "complex data"() -> (w166:cdb[])
            n75 = case shown="\"No\"" "Subtract a circle?" {
              tunnel: w169 -> [w207 _]
              tunnel: [w198 w215] -> w168
              tunnel: w166 -> [w197 w215]
              frame "Yes", Default {
                w212 = cursor_action."range" ("cursor action")
                n76 = call "replace cursor - plot ref - V2.vi"("Plot ref in"=w207, "cursor index"=0, "cursor action"=w212) -> ("read X"=w211:dbl, "read Y"=w210:dbl)  [unwired: 14 in, 1 out]
                n77 = call "replace cursor - plot ref - V2.vi"("Plot ref in"=w207, "cursor index"=1, "cursor action"=w212) -> ("read X"=w209:dbl, "read Y"=w208:dbl)  [unwired: 14 in, 1 out]
                n78 = Re/Im To Complex(1:w210, 2:w211) -> (0:w204:cdb)
                n79 = Re/Im To Complex(1:w208, 2:w209) -> (0:w206:cdb)
                n80 = Subtract(x=w206, y=w204) -> (x-y=w205:cdb)
                n81 = Subtract(x=w197, y=w204) -> (x-y=w203:cdb[])
                n82 = Complex To Polar(r * e^(i*theta)=w205) -> (r=w201:dbl)  [unwired: 1 out]
                n83 = Complex To Polar(r * e^(i*theta)=w203) -> (r=w202:dbl[])  [unwired: 1 out]
                n84 = Divide(x=w202, y=w201) -> (x/y=w200:dbl[])
                n85 = Divide(x=w197, y=w200) -> (x/y=w199:cdb[])
                n86 = Subtract(x=w197, y=w199) -> (x-y=w198:cdb[])
              }
              frame "No" {
              }
            }
            n87 = local read "chunks"() -> (w174:T12)
            n88 = Unbundle By Name(w174) -> ("update rate (Hz)"=w176:dbl)
            n89 = Multiply(x="highlight last # sec", y=w176) -> (x*y=w177:dbl)
            n90 = Round Toward -Infinity(1:w177) -> (0:w178:dbl)
            n91 = To Long Integer(number=w178) -> (32bit integer=w172:i32)
            n92 = Subtract(x=w165, y=w172) -> (x-y=w171:i32)
            n93 = Array Subset(array=w166, index=w171, length=w172) -> (w185:cdb[])
            n94 = local read "frequency"() -> (w173:dbl[])
            n95 = Array Subset(array=w168, length=w165) -> (w183:cdb[])  [unwired: 1 in]
            n96 = Array Subset(array=w166, length=w165) -> (w167:cdb[])  [unwired: 1 in]
            n97 = Complex To Re/Im(x + iy=w185) -> (x=w186:dbl[], y=w187:dbl[])
            n98 = Complex To Re/Im(x + iy=w183) -> (x=w191:dbl[], y=w192:dbl[])
            n99 = Complex To Re/Im(x + iy=w167) -> (x=w164:dbl[], y=w163:dbl[])
            n100 = Divide(x=w173, y=1000 ("dimension size")) -> (x/y=w189:dbl[])
            n101 = local read "line one"() -> (w195:cluster{dbl[], dbl[]})
            n102 = local read "circle"() -> (w194:cluster{dbl[], dbl[]})
            n103 = local read "line two"() -> (w196:cluster{dbl[], dbl[]})
            n104 = local read "fancy lines"() -> (w193:cluster{dbl[], dbl[]}[])
            n105 = Bundle(w189, w191) -> (w179:cluster{dbl[], dbl[]})  [unwired: 1 out]
            n106 = Bundle(w189, w192) -> (w181:cluster{dbl[], dbl[]})  [unwired: 1 out]
            n107 = Bundle(w164, w163) -> (w184:cluster{dbl[], dbl[]})  [unwired: 1 out]
            n108 = Bundle(w186, w187) -> (w188:cluster{dbl[], dbl[]})  [unwired: 1 out]
            n109 = Build Array (concatenate)(w179, w181, w193) -> (→"Plot:response":cluster{dbl[], dbl[]}[])
            n110 = Build Array(w184, w188, w194, w195, w196) -> (→"Plot:complex plane":cluster{dbl[], dbl[]}[])
          }
        }
      }
      event "complex plane scale gauge": Value Change {
        n111 = event-data() -> ()  [unwired: 1 in, 1 out]
        n112 = Generate User Event(user event=w216, event data cluster="scale gauge changed" ("event data")) -> ()  [unwired: 2 in, 2 out]
      }
      event "Plot:complex plane": Cursor Move {
        n113 = event-data() -> ()  [unwired: 1 in, 5 out]
        n114 = Generate User Event(user event=w218, event data cluster="draw circle" ("event data")) -> ()  [unwired: 2 in, 2 out]
      }
      event "show plot pallets": Value Change {
        n115 = event-data() -> ("NewVal"=w221:bool)  [unwired: 1 in]
        n116 = property on="Property Node" class="XYGraph (strict)"(reference=w222, "ScaleLegendVis"=w221, "Palette Visible"=w221, "Legend Visible"=w221) -> ()  [unwired: 1 in, 2 out]
        n117 = property on="Property Node" class="XYGraph (strict)"(reference=w220, "ScaleLegendVis"=w221, "Palette Visible"=w221, "Legend Visible"=w221) -> ()  [unwired: 1 in, 2 out]
      }
    }
  }
  n118 = while {
    tunnel: w70 -> [w235]
    shift-right: [w233] -> w91
    shift-left: w96 -> [w232]
    shift-right: [w229] -> _
    shift-left: w78 -> [w231]
    tunnel: "Graph update rate, ms" -> [w230]
    shift-right: [w227] -> w59
    shift-left: 0 ("disabled index (col)") -> [w228]
    shift-right: [w225] -> w60
    shift-left: w64 -> [w226]
    tunnel: w3 -> [w224]
    tunnel: w1 -> [w223]
    stop <- w234 stop-if-true
    # "dispatch loop"
    n119 = event shown="[1] <New data>: User Event" {
      selector: w235 -> [_ _ _]
      dyn-events: _ -> [_ _ _]
      timeout: _ -> [_ _ _]
      tunnel: [_ _ TRUE] -> w234
      tunnel: [w239 w257 w274] -> w233
      tunnel: w232 -> [w239 w258 w274]
      tunnel: w231 -> [w238 w254 w273]
      tunnel: w230 -> [_ w252 _]
      tunnel: [w238 w260 w273] -> w229
      tunnel: w228 -> [w237 w246 w272]
      tunnel: [w237 w243 w272] -> w227
      tunnel: w226 -> [w236 w248 w271]
      tunnel: [w236 w247 w271] -> w225
      tunnel: w224 -> [_ _ _]
      tunnel: w223 -> [_ w240 w269]
      event Timeout {
        n120 = event-data() -> ()  [unwired: 3 out]
      }
      event User Event {
        # "complex data"
        # "frequency"
        # "Plot data"
        # "New data arrives as a 2D complex array. Two rows are: \n1. frequency (as a complex number) ........... \n2. complex response .............."
        # "Insert new data"
        n121 = event-data() -> ("New data"=w251:cdb[][])  [unwired: 1 out]
        n122 = Tick Count (ms)() -> (millisecond timer value=w253:u32)
        n123 = Index Array(array=w251, index (row) #1=0 ("disabled index (col)"), index (row) #2=1 ("disabled index (col)")) -> (element #1=w245:cdb[], element #2=w242:cdb[])  [unwired: 2 in]
        n124 = Complex To Re/Im(x + iy=w245) -> (x=w244:dbl[])  [unwired: 1 out]
        n125 = Replace Array Subset(array=w248, new element=w244, index=w246) -> (w247:dbl[])
        "frequency" <- w247
        n126 = Replace Array Subset(array=w258, new element=w242, index=w246) -> (w257:cdb[])
        "complex data" <- w257
        n127 = Array Size(array=w242) -> (size(s)=w241:i32)
        n128 = Less?(x=w254, y=w253) -> (x < y?=w256:bool)
        n129 = Add(x=w241, y=w246) -> (x+y=w243:i32)
        "#data points so far" <- w243
        n130 = And(x=w256, y="Plot when running") -> (x .and. y?=w259:bool)
        n131 = case shown="True" w259 {
          tunnel: w257 -> [_ _]
          tunnel: w253 -> [_ w265]
          tunnel: [w261 w264] -> w260
          tunnel: w254 -> [w261 _]
          tunnel: w247 -> [_ _]
          tunnel: w252 -> [_ w266]
          tunnel: w240 -> [_ w262]
          frame False {
          }
          frame True {
            n132 = Add(x=w266, y=w265) -> (x+y=w264:u32)
            n133 = Generate User Event(user event=w262, event data cluster="plot all" ("event data")) -> ()  [unwired: 2 in, 2 out]
          }
        }
      }
      event User Event {
        n134 = event-data() -> ()  [unwired: 2 out]
        n135 = Generate User Event(user event=w269, event data cluster="plot all" ("event data")) -> (user event out=w268:refnum<user-event>)  [unwired: 2 in, 1 out]
        n136 = Generate User Event(user event=w268, event data cluster="stop" ("event data")) -> ()  [unwired: 2 in, 2 out]
      }
    }
  }
  n137 = for {
    N: w85 -> [w327]
    tunnel: w50 -> [w329]
    tunnel: [w299] -> w97
    tunnel: w94 -> [w323]
    tunnel: w51 -> [w330]
    tunnel: ["stop"] -> w90
    shift-right: [w318] -> w61
    shift-left: w46 -> [w320]
    tunnel: w41 -> [w319]
    shift-right: [w313] -> w72
    shift-left: _ -> [_]
    shift-right: [w284] -> _
    shift-left: w45 -> [w315]
    shift-right: [w287] -> w38
    shift-left: w40 -> [w288]
    shift-right: [w317] -> _
    shift-left: w39 -> [w289]
    shift-right: [w302] -> _
    shift-left: w42 -> [w316]
    shift-right: [w314] -> w71
    shift-left: _ -> [_]
    tunnel: w68 -> [w311]
    shift-right: [w294] -> _
    shift-left: _ -> [_]
    shift-right: [w293] -> _
    shift-left: _ -> [w295]
    shift-right: [w290] -> _
    shift-left: w35 -> [w286]
    shift-left: w34 -> [_]
    shift-left: w10 -> [w282]
    tunnel: w11 -> [w281]
    i -> [w299]
    stop <- w332 stop-if-true
    (unwired) next_chunk_--_action."next chunk - peaks are known" ("next chunk action")
    w291 = FALSE  # first time ?
    (unwired) 1 ("length")
    (unwired) 1 ("index")
    w312 = FALSE  # first time ?
    # "build 2D array { freq; complex response}"
    # "Data aquisition loop"
    n138 = Less?(x=w323, y=w299) -> (x < y?=w331:bool)
    n139 = Equal To 0?(x=w299) -> ()  [unwired: 1 out]
    n140 = Divide(x=w299, y=w327) -> (x/y=w326:dbl)
    n141 = case shown="True" w331 {
      tunnel: w330 -> [_ w340]
      tunnel: w329 -> [_ w335]
      tunnel: w299 -> [_ w334]
      tunnel: w320 -> [w333 w338]
      tunnel: [w333 w336] -> w328
      frame False {
      }
      frame True {
        # "Round down  last read"
        n142 = Multiply(x=w335, y=w334) -> (x*y=w339:i32)
        n143 = Subtract(x=w340, y=w339) -> (x-y=w337:i32)
        n144 = Bundle By Name(cluster=w338, "Samples per read"=w337) -> (w336:T13)
      }
    }
    n145 = Re/Im To Complex(1:0.0, 2:w282) -> (0:w304:cdb[])
    n146 = Build Array(w304, w286) -> (w303:cdb[][])
    n147 = Multiply(x=w326, y=100.0) -> (x*y=→"Progress, %":dbl)
    n148 = Generate User Event(user event=w311, event data cluster=w303) -> ()  [unwired: 2 in, 2 out]
    n149 = Unbundle By Name(w328) -> ()  [unwired: 2 out]
    n150 = call "single sweep - upload freq window.vi"("first time ?"=w312, "timeout"=w319, "error in (no error)"=w288, "F-window array"=w289, "task in"=w315, "RUS settings"=w320) -> ("error out"=w283:errorcluster, "task out"=w284:refnum<k21>, "RUS settings out"=w318:T13, "DO array  making time"=w313:u32, "DO write time"=w314:u32)  [unwired: 1 in]
    n151 = call "NI-DAQ RUS Lockin.vi"("Init?"=w291, "error in (no error)"=w288, "RUS settings"=w328) -> ("error out"=w285:errorcluster, "AvailSampPerChan"=w292:u32, "Lockin out"=w310:dbl[][])  [unwired: 5 in, 1 out]
    n152 = Merge Errors(w285, w283) -> (w287:errorcluster)
    n153 = local write "Samples in buffer"(w292) -> ()
    n154 = local read "adaptive state"() -> (w301:T8)
    n155 = call "next chunk - V4.vi"("next chunk action"=w281, "x + iy"=w286, "chunks"=w316, "F Array in"=w282) -> ("chunks out"=w280:T12, "F Array out"=w317:dbl[], "fancy lines"=→"fancy lines":cluster{dbl[], dbl[]}[], "fancy circles"=→"fancy circles":cluster{dbl[], dbl[]}[])  [unwired: 4 in]
    n156 = Unbundle By Name(w280) -> ("adaptive parameters.peaks are known -- parameters.near omega (kHz)"=→"near omega (kHz)":dbl, "adaptive parameters.peaks are known -- parameters.near gamma (kHz)"=→"near gamma (kHz)":dbl)
    n157 = Bundle By Name(cluster=w280, "adaptive parameters"=w301) -> (w302:T12)
    n158 = Tick Count (ms)() -> (millisecond timer value=w298:u32)
    n159 = Index Array(array=w310, index (row) #1=0 ("index"), index (row) #2=1 ("length")) -> (element #1=w307:dbl[], element #2=w306:dbl[])  [unwired: 2 in]
    n160 = Divide(x=w298, y=u32 1000) -> (x/y=w294:dbl)
    n161 = Equal To 0?(x=w299) -> (x = 0?=w296:bool)
    n162 = Re/Im To Complex(1:w306, 2:w307) -> (0:w290:cdb[])
    "last data" <- w290
    n163 = local write "chunks"(w302) -> ()
    n164 = Select(t=w294, s=w296, f=w295) -> (s? t:f=w293:dbl)
    n165 = Unbundle By Name(w287) -> ("status"=w321:bool)
    n166 = Subtract(x=w294, y=w293) -> (x-y=w300:dbl)
    n167 = local write "progress (sec)"(w300) -> ()
    n168 = Compound Arithmetic op=OR("stop", w321) -> (w332:bool)
  }
  "Loop counter" <- w97
  "DO array  making time" <- w72
  "DO write time, ms" <- w71
  n169 = Increment(x=w97) -> (x+1=w93:i32)
  n170 = Divide(x=w93, y=w98) -> (x/y=w101:dbl)
  n171 = Multiply(x=w101, y=100.0) -> (x*y=w99:dbl)
  n172 = local write "Progress, %"(w99) -> ()
  n173 = disable-structure shown="Disabled" {
    frame Disabled {
      n174 = Unbundle By Name() -> ("Lockin mode"=w341:enum16{"SRS", "NI-DAQ"})  [unwired: 1 in]
      n175 = case shown="\"NI-DAQ\"" w341 {
        tunnel: [_ w343] -> _
        tunnel: [_ w342] -> _
        frame "SRS", Default {
        }
        frame "NI-DAQ" {
          # "Download freq array"
          n176 = call "ProgramFreqBulk.vi"() -> ("error out"=w343:errorcluster, "RUS settings out"=w342:T13)  [unwired: 5 in, 5 out]
        }
      }
    }
    frame Enabled {
    }
  }
  n177 = Unbundle By Name("sweep settings") -> ("Zero signal?"=w7:bool, "save freq units"=w6:enum16{"kHz", "Hz"}, "Bypass error dialog"=w8:bool)
  n178 = Array Subset(array=w60, length=w59) -> (w52:dbl[])  [unwired: 1 in]
  n179 = Array Subset(array=w91, length=w59) -> (w63:cdb[])  [unwired: 1 in]
  n180 = call "single sweep - rus clean up.vi"("Zero amplitude at the end"=w7, "Stop user event"=w62, "error in (no error)"=w38, "RUS settings"=w61) -> ("error out"=w86:errorcluster, "STD status byte"=→"STD status byte":u8, "Error status byte\n(bit 5 - FAST aborted)"=→"Error status byte\n(bit 5 - FAST aborted)":u8, "RUS settings out"=w81:T13)  [unwired: 4 in]
  n181 = Not(x=w90) -> (.not. x?=w79:bool)
  n182 = disable-structure shown="Enabled" {
    disable-tunnel: w63 -> [w353 _]
    disable-tunnel: w52 -> [w346 _]
    frame Disabled {
      n183 = Complex To Re/Im(x + iy=w353) -> (x=w352:dbl[], y=w351:dbl[])
      n184 = disable-structure shown="Enabled" {
        disable-tunnel: w351 -> [w361 w363]
        disable-tunnel: w352 -> [w360 w362]
        disable-tunnel: [w359 w362] -> w349
        disable-tunnel: [w358 w363] -> w348
        disable-tunnel: _ -> [w357 _]
        frame Disabled {
          n185 = call "Rotate Lockin Phase.vi"("Phase"=w357, "Array Y in"=w361, "Array X in"=w360) -> ("Array Y out"=w358:dbl[], "Array X out"=w359:dbl[])  [unwired: 7 out]
        }
        frame Enabled {
        }
      }
      n186 = Divide(x=w346, y=1000 ("dimension size")) -> (x/y=w345:dbl[])
      n187 = Bundle(w349, w348) -> (w350:cluster{dbl[], dbl[]})  [unwired: 1 out]
      n188 = Bundle(w345, w349) -> (w356:cluster{dbl[], dbl[]})  [unwired: 1 out]
      n189 = Bundle(w345, w348) -> (w355:cluster{dbl[], dbl[]})  [unwired: 1 out]
      n190 = Build Array(w356, w355) -> (w354:cluster{dbl[], dbl[]}[])
      n191 = Build Array(w350) -> (w347:cluster{dbl[], dbl[]}[])
      n192 = local write "Plot:complex plane"(w347) -> ()
      n193 = local write "Plot:response"(w354) -> ()
    }
    frame Enabled {
    }
  }
  n194 = case shown="True" w79 {
    tunnel: w86 -> [w364 w371]
    tunnel: [w364 w369] -> w103
    tunnel: w63 -> [_ w366]
    tunnel: w81 -> [_ w368]
    tunnel: w52 -> [_ w367]
    tunnel: w6 -> [_ w365]
    frame False {
    }
    frame True {
      n195 = call "single sweep - save rus data.vi"("save freq units"=w365, "error in (no error)"=w371, "rus response"=w366, "F Array"=w367, "RUS settings"=w368) -> ("error out"=w369:errorcluster, "Actual file path"=→"Actual file path":path)  [unwired: 5 in]
    }
  }
  n196 = disable-structure shown="Disabled" {
    frame Disabled {
      n197 = while {
        shift-right: [w375] -> _
        shift-left: _ -> [w376]
        shift-right: [w374] -> _
        shift-left: _ -> [w377]
        tunnel: [w372] -> _
        stop <- TRUE stop-if-true
        n198 = property class="DAQmx Write"(reference=w376, error in=w377) -> (reference out=w375:refnum<k21>, error out=w374:errorcluster, "SpaceAvail"=w372:u32)
      }
    }
    frame Enabled {
    }
  }
  n199 = case shown="False" w8 {
    tunnel: [w379 w381] -> w106
    tunnel: w103 -> [w378 w381]
    frame False {
      w380 = T19 3 items=["no dialog", "OK message", "continue or stop message", "OK message + warnings", "continue/stop + warnings"] ("type of dialog (OK msg:1)")
      n200 = call <vilib>:"General Error Handler.vi"("type of dialog (OK msg:1)"=w380, "error in (no error)"=w378) -> ("error out"=w379:errorcluster)  [unwired: 1 in, 12 out]
    }
    frame True {
    }
  }
  "error out" <- w106
